vi "Robot_SpeedTest.vi"   [LabVIEW 2012]
uses:
  Messages.ctl
  Support VIs/messageTypes.ctl
  Support VIs/speeds.ctl
  StopTDef.ctl
  <vilib>/robotics/Starter Kit/2.0/9632 Host Interface/NI_Robotics_Starter Kit Host_9632_2.0.lvclass
  <vilib>/robotics/Starter Kit/Host Interface/NI_Robotics_Starter Kit Host.lvclass
types:
  T1 = typedef "speeds.ctl" = cluster{"left motor [rad/s]":dbl, "right motor [rad/s]":dbl}
  T2 = typedef "Messages.ctl" = cluster{"message data":variant, "message type":T3}
  T3 = typedef "messageTypes.ctl" = enum16{"Speeds", "Stop", "PolarCoordinates", "Gains", "Setpoints"}
  T4 = typedef "StopTDef.ctl" = cluster{"stop":bool}
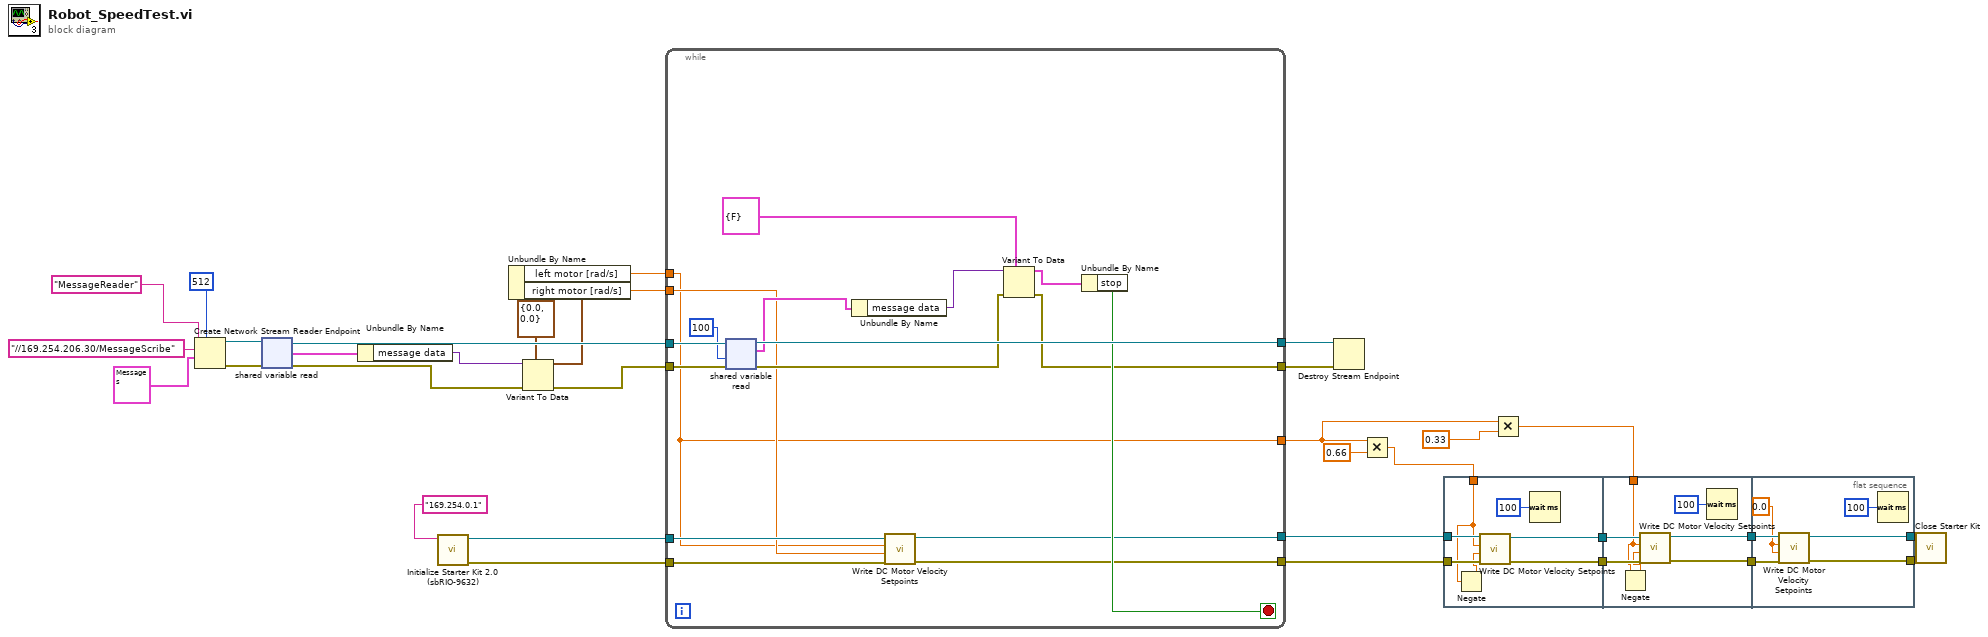
[diagram p0: block diagram]
diagram:
  n1 = Create Network Stream Reader Endpoint(7:512 ("reader buffer size"), 9:T2 {"message data"=variant, "message type"=enum."Setpoints"} ("message"), 10:"//169.254.206.30/MessageScribe" ("writer url"), 11:"MessageReader" ("reader name")) -> (0:w27:errorcluster, 3:w28:refnum<k21>)  [unwired: 3 in]
  n2 = shared-variable-read(w28, w27) -> (w26:refnum<k21>, w24:errorcluster, w13:T2)  [unwired: 1 in, 1 out]
  n3 = Unbundle By Name(w13) -> ("message data"=w12:variant)
  n4 = call <vilib>:"Initialize Starter Kit 2.0 (sbRIO-9632).vi"("IP address (\"\")"="169.254.0.1" ("IP address (\"\")")) -> ("error out"=w10:errorcluster, "FPGA starter kit host 2.0 out"=w11:refnum<class "NI_Robotics_Starter Kit Host_9632_2.0.lvclass">)  [unwired: 9 in]
  n5 = Variant To Data(error in=w24, type=T1 {"left motor [rad/s]"=0.0, "right motor [rad/s]"=0.0} ("Speeds"), Variant=w12) -> (data=w22:T1, error out=w23:errorcluster)
  n6 = Unbundle By Name(w22) -> ("left motor [rad/s]"=w21:dbl, "right motor [rad/s]"=w20:dbl)
  n7 = while {
    tunnel: w11 -> [w50]
    tunnel: w10 -> [w49]
    tunnel: w26 -> [w48]
    tunnel: w23 -> [w47]
    tunnel: w21 -> [w34]
    tunnel: w20 -> [w35]
    tunnel: [w38] -> w17
    tunnel: [w37] -> w16
    tunnel: [w46] -> w19
    tunnel: [w39] -> w18
    tunnel: [w34] -> w2
    stop <- w40 stop-if-true
    n8 = shared-variable-read(w48, w47, 100 ("timeout ms (-1)")) -> (w46:refnum<k21>, w42:errorcluster, w45:T2)  [unwired: 1 out]
    n9 = Unbundle By Name(w45) -> ("message data"=w44:variant)
    n10 = call <vilib>:"Write DC Motor Velocity Setpoints.vi"("error in (no error)"=w49, "right motor ccw velocity (rad/s)"=w35, "left motor ccw velocity (rad/s)"=w34, "starter kit host in"=w50) -> ("error out"=w37:errorcluster, "starter kit host out"=w38:refnum<class "NI_Robotics_Starter Kit Host_9632_2.0.lvclass">)  [unwired: 6 in]
    n11 = Variant To Data(error in=w42, type=T4 {"stop"=FALSE}, Variant=w44) -> (data=w41:T4, error out=w39:errorcluster)
    n12 = Unbundle By Name(w41) -> ("stop"=w40:bool)
  }
  n13 = Destroy Stream Endpoint(8:w18, 11:w19) -> ()  [unwired: 1 out]
  n14 = Multiply(x=w2, y=0.66) -> (x*y=w4:dbl)
  n15 = flat-sequence {
    tunnel: w16 -> [w56]
    tunnel: w17 -> [w57]
    tunnel: [w55] -> w7
    tunnel: [w54] -> w6
    tunnel: w4 -> [w52]
    tunnel: [w64] -> w9
    tunnel: [w63] -> w8
    tunnel: w7 -> [w62]
    tunnel: w6 -> [w61]
    tunnel: w1 -> [w59]
    tunnel: [w67] -> w15
    tunnel: [w66] -> w14
    tunnel: w9 -> [w70]
    tunnel: w8 -> [w69]
    frame #0 {
      n16 = Negate(x=w52) -> (-x=w53:dbl)
      n17 = call <vilib>:"Write DC Motor Velocity Setpoints.vi"("error in (no error)"=w56, "right motor ccw velocity (rad/s)"=w53, "left motor ccw velocity (rad/s)"=w52, "starter kit host in"=w57) -> ("error out"=w54:errorcluster, "starter kit host out"=w55:refnum<class "NI_Robotics_Starter Kit Host_9632_2.0.lvclass">)  [unwired: 6 in]
      n18 = Wait (ms)(milliseconds to wait=u32 100) -> ()  [unwired: 1 out]
    }
    frame #1 {
      n19 = Negate(x=w59) -> (-x=w60:dbl)
      n20 = call <vilib>:"Write DC Motor Velocity Setpoints.vi"("error in (no error)"=w61, "right motor ccw velocity (rad/s)"=w60, "left motor ccw velocity (rad/s)"=w59, "starter kit host in"=w62) -> ("error out"=w63:errorcluster, "starter kit host out"=w64:refnum<class "NI_Robotics_Starter Kit Host_9632_2.0.lvclass">)  [unwired: 6 in]
      n21 = Wait (ms)(milliseconds to wait=u32 100) -> ()  [unwired: 1 out]
    }
    frame #2 {
      w68 = 0.0
      n22 = call <vilib>:"Write DC Motor Velocity Setpoints.vi"("error in (no error)"=w69, "right motor ccw velocity (rad/s)"=w68, "left motor ccw velocity (rad/s)"=w68, "starter kit host in"=w70) -> ("error out"=w66:errorcluster, "starter kit host out"=w67:refnum<class "NI_Robotics_Starter Kit Host_9632_2.0.lvclass">)  [unwired: 6 in]
      n23 = Wait (ms)(milliseconds to wait=u32 100) -> ()  [unwired: 1 out]
    }
  }
  n24 = Multiply(x=w2, y=0.33) -> (x*y=w1:dbl)
  n25 = call-dynamic "Close Starter Kit.vi"("error in (no error)"=w14, "starter kit host in"=w15) -> ()  [unwired: 9 in, 1 out]
